vi "smu-dmm-test.vi"() -> ()   [LabVIEW 2020]
uses:
  Realization/NI DMM/NI DMM.lvclass
  Realization/NI DMM/TypeDefs/DMM waveform settings.ctl
  <instrlib>/niDMM/nidmm.llb/niDMM Waveform Function.ctl
  Realization/NI DMM/TypeDefs/Trigger settings.ctl
  <instrlib>/niDMM/nidmm.llb/niDMM Trigger.ctl
  <instrlib>/niDMM/nidmm.llb/niDMM Slope.ctl
  Realization/PIPX40 Relay/PIPX40 Relay.lvclass
  Realization/PIPX40 Matrix/PIPX40 Matrix.lvclass
  <instrlib>/niDCPower/nidcpower.llb/niDCPower Source Mode.ctl
  <instrlib>/niDCPower/nidcpower.llb/niDCPower Wait For Event - Event.ctl
  <instrlib>/niDCPower/nidcpower.llb/niDCPower Output Function.ctl
panel:
  in  "current limit range":dbl=0.01 format="%.6p"
  in  "voltage level range":dbl=6.0 format="%.6p"
  in  "current limit":dbl=0.01 format="%.6p"
  in  "voltage level":dbl=2.0 format="%.6p"
  in  "Source:Advanced:Source Delay":dbl=0.1
  out "Voltage Measurement":dbl
  out "Current Measurement":dbl
  out "Compliance/Limit Reached":bool
  in  "Channel Name":string="0"
  in  "Resource Name":refnum<k15>="NI_SMU1"
  out "relay info":variant
  out "Waveform Graph":dynamicdata(graph)
  out "error out":errorcluster
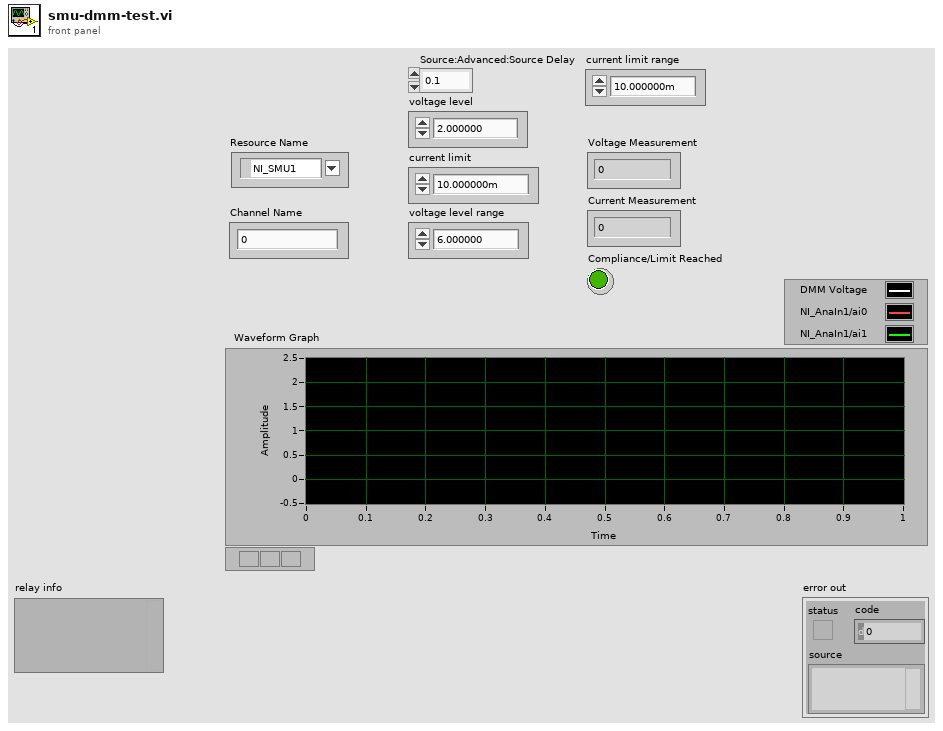
[diagram p1: front panel]
types:
  T1 = typedef "niDCPower Output Function.ctl" = i32
  T2 = typedef "niDCPower Wait For Event - Event.ctl" = i32
  T3 = typedef "niDCPower Source Mode.ctl" = i32
  T4 = typedef "NI DMM.lvlib/NI DMM.lvclass/Trigger settings.ctl" = cluster{"Trigger Source":T5, "Trigger Delay (sec)":dbl, "Slope":T6}
  T5 = typedef "niDMM Trigger.ctl" = enum16{"Immediate", "External", "TTL 0", "TTL 1", "TTL 2", "TTL 3", "TTL 4", "TTL 5", "TTL 6", "Software", "TTL 7", "PXI Star", "LBR Trig 1", "Aux Trig 1"}
  T6 = typedef "niDMM Slope.ctl" = enum16{"Rising Edge", "Falling Edge"}
  T7 = typedef "NI DMM.lvlib/NI DMM.lvclass/DMM waveform settings.ctl" = cluster{"Waveform Points":i32, "Function":T8, "Rate":dbl, "Range":dbl, "Settle Time":dbl}
  T8 = typedef "niDMM Waveform Function.ctl" = i32
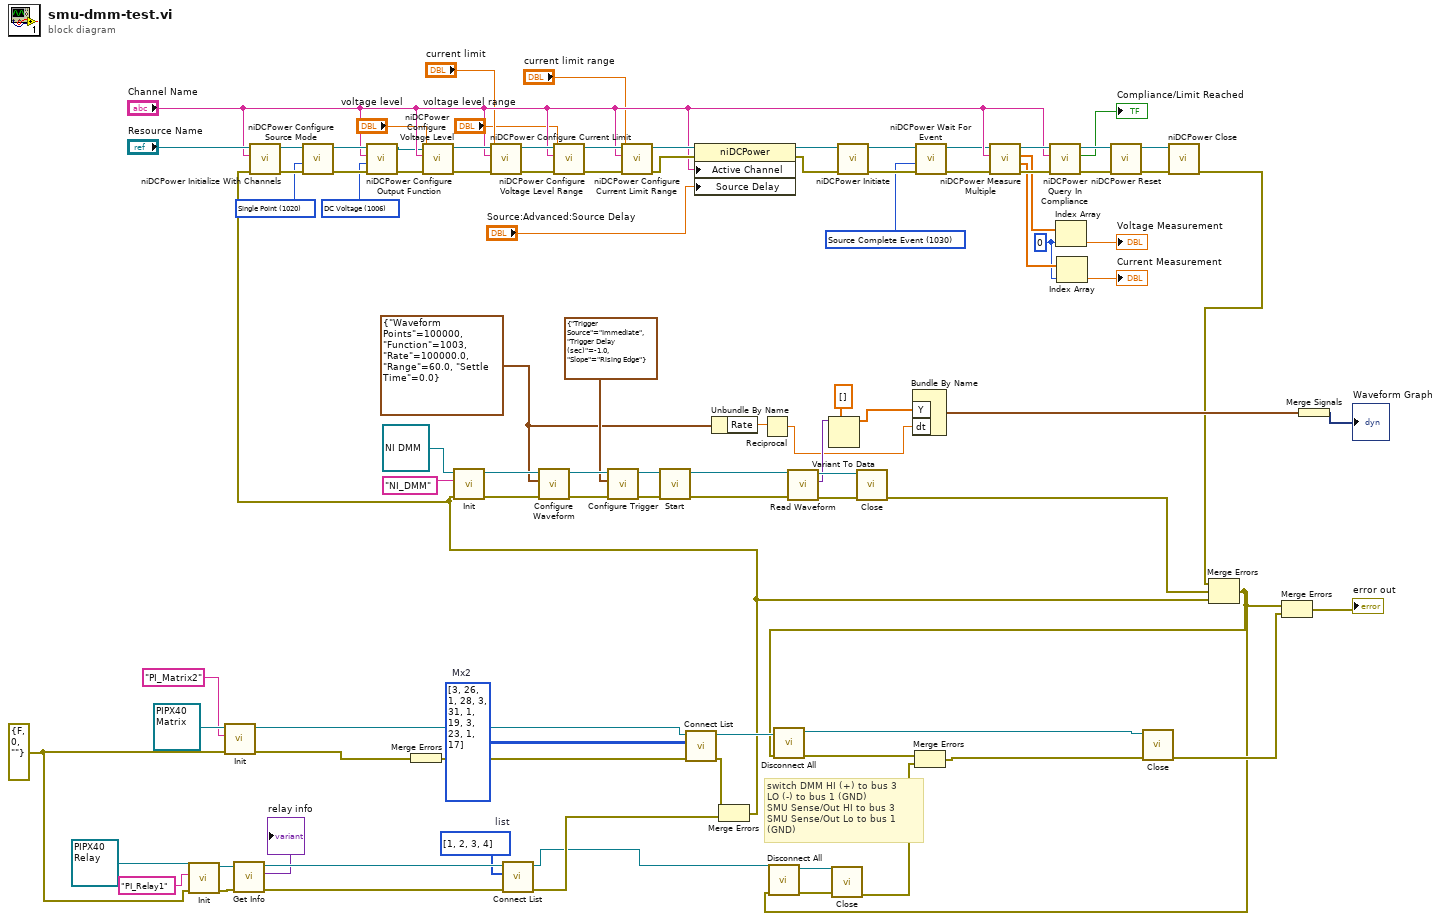
[diagram p0: block diagram]
diagram:
  w12 = T1 1006 items=["DC Voltage"=1006, "DC Current"=1007, "Pulse Voltage"=1049, "Pulse Current"=1050] ("output function")
  w16 = T2 1030 items=["Source Complete Event"=1030, "Measure Complete Event"=1031, "Sequence Iteration Complete Event"=1032, "Sequence Engine Done Event"=1033] ("event")
  w28 = 0 ("index")
  w37 = T3 1020 items=["Single Point"=1020, "Sequence"=1021] ("source mode")
  w59 = i32[] [1, 2, 3, 4]  # list
  w73 = T7 {"Waveform Points"=100000, "Function"=1003, "Rate"=100000.0, "Range"=60.0, "Settle Time"=0.0}
  w58 = errorcluster {"status"=FALSE, "code"=0, "source"=""} ("error in (no error)")
  w93 = i32[][] [[3, 26], [1, 28], [3, 31], [1, 19], [3, 23], [1, 17]]  # Mx2
  # "switch DMM HI (+) to bus 3 \nLO (-) to bus 1 (GND)\nSMU Sense/Out HI to bus 3\nSMU Sense/Out Lo to bus 1 (GND)"
  n1 = call-dynamic "Init.vi"("error in (no error)"=w58, "Params"="PI_Relay1" ("String"), "PIPXI40 Base in"=refnum<class "PIPX40 Relay.lvclass"> refnum ("Pickering.lvlib:PIPX40 Relay.lvclass")) -> ("error out"=w68:errorcluster, "PIPXI40 Base out"=w65:refnum<class "PIPX40 Relay.lvclass">)  [unwired: 7 in]
  n2 = call-dynamic "Init.vi"("error in (no error)"=w58, "Params"="PI_Matrix2" ("String"), "PIPXI40 Base in"=refnum<class "PIPX40 Matrix.lvclass"> refnum ("PIPXI40 Matrix in")) -> ("error out"=w53:errorcluster, "PIPXI40 Base out"=w51:refnum<class "PIPX40 Matrix.lvclass">)  [unwired: 7 in]
  n3 = call-dynamic "Get Info.vi"("error in (no error)"=w68, "PIPXI40 Base in"=w65) -> ("error out"=w62:errorcluster, "Info"=→"relay info":variant, "PIPXI40 Base out"=w64:refnum<class "PIPX40 Relay.lvclass">)  [unwired: 7 in]
  n4 = Merge Errors(w53) -> (w86:errorcluster)
  n5 = call-dynamic "Connect List.vi"("error in (no error)"=w62, "Params"=w59, "PIPXI40 Switching in"=w64) -> ("error out"=w55:errorcluster, "PIPXI40 Switching out"=w54:refnum<class "PIPX40 Relay.lvclass">)  [unwired: 7 in]
  n6 = call-dynamic "Connect List.vi"("error in (no error)"=w86, "Params"=w93, "PIPXI40 Matrix in"=w51) -> ("error out"=w89:errorcluster, "PIPXI40 Matrix out"=w92:refnum<class "PIPX40 Matrix.lvclass">)  [unwired: 7 in]
  n7 = Unbundle By Name(w73) -> ("Rate"=w72:dbl)
  n8 = Merge Errors(w89, w55) -> (w1:errorcluster)
  n9 = call <instrlib>:"niDCPower Initialize With Channels.vi"("error in (no error)"=w1, "channels"="Channel Name", "resource name"="Resource Name") -> ("error out"=w41:errorcluster, "instrument handle out"=w40:refnum<k15>)  [unwired: 2 in, 5 out]
  n10 = call <instrlib>:"niDCPower Configure Source Mode.vi"("error in (no error)"=w41, "source mode"=w37, "instrument handle"=w40) -> ("error out"=w39:errorcluster, "instrument handle out"=w38:refnum<k15>)  [unwired: 7 out]
  n11 = call <instrlib>:"niDCPower Configure Output Function.vi"("error in (no error)"=w39, "output function"=w12, "channel name"="Channel Name", "instrument handle"=w38) -> ("error out"=w14:errorcluster, "instrument handle out"=w15:refnum<k15>)  [unwired: 6 out]
  n12 = call <instrlib>:"niDCPower Configure Voltage Level.vi"("error in (no error)"=w14, "voltage level"="voltage level", "channel name"="Channel Name", "instrument handle"=w15) -> ("error out"=w46:errorcluster, "instrument handle out"=w47:refnum<k15>)  [unwired: 6 out]
  n13 = call-dynamic "Init.vi"("error in (no error)"=w1, "Params"="NI_DMM", "NI DMM in"=refnum<class "NI DMM.lvclass"> refnum) -> ("error out"=w84:errorcluster, "NI DMM out"=w85:refnum<class "NI DMM.lvclass">)  [unwired: 7 in]
  n14 = call <instrlib>:"niDCPower Configure Current Limit.vi"("error in (no error)"=w46, "current limit"="current limit", "channel name"="Channel Name", "instrument handle"=w47) -> ("error out"=w36:errorcluster, "instrument handle out"=w35:refnum<k15>)  [unwired: 1 in, 5 out]
  n15 = call-dynamic "Configure Waveform.vi"("error in (no error)"=w84, "Params"=w73, "NI DMM in"=w85) -> ("error out"=w80:errorcluster, "NI DMM out"=w81:refnum<class "NI DMM.lvclass">)  [unwired: 7 in]
  n16 = call <instrlib>:"niDCPower Configure Voltage Level Range.vi"("error in (no error)"=w36, "voltage level range"="voltage level range", "channel name"="Channel Name", "instrument handle"=w35) -> ("error out"=w34:errorcluster, "instrument handle out"=w33:refnum<k15>)  [unwired: 6 out]
  n17 = call-dynamic "Configure Trigger.vi"("error in (no error)"=w80, "Params"=T4 {"Trigger Source"=enum."Immediate", "Trigger Delay (sec)"=-1.0, "Slope"=enum."Rising Edge"}, "NI DMM in"=w81) -> ("error out"=w5:errorcluster, "NI DMM out"=w4:refnum<class "NI DMM.lvclass">)  [unwired: 7 in]
  n18 = call <instrlib>:"niDCPower Configure Current Limit Range.vi"("error in (no error)"=w34, "current limit range"="current limit range", "channel name"="Channel Name", "instrument handle"=w33) -> ("error out"=w22:errorcluster, "instrument handle out"=w25:refnum<k15>)  [unwired: 6 out]
  n19 = call-dynamic "Start.vi"("error in (no error)"=w5, "DMM in"=w4) -> ("error out"=w2:errorcluster, "DMM out"=w3:refnum<class "NI DMM.lvclass">)  [unwired: 8 in]
  n20 = property class="niDCPower"(reference=w25, error in=w22, "Active Channel"="Channel Name", "Source Delay"="Source:Advanced:Source Delay") -> (reference out=w24:refnum<k15>, error out=w23:errorcluster)
  n21 = Reciprocal(x=w72) -> (1/x=w71:dbl)
  n22 = call-dynamic "Read Waveform.vi"("error in (no error)"=w2, "NI DMM in"=w3) -> ("error out"=w78:errorcluster, "Data"=w76:variant, "NI DMM out"=w77:refnum<class "NI DMM.lvclass">)  [unwired: 7 in]
  n23 = Variant To Data(type=dbl[] [], Variant=w76) -> (data=w74:dbl[])  [unwired: 1 in, 1 out]
  n24 = call <instrlib>:"niDCPower Initiate.vi"("error in (no error)"=w23, "instrument handle"=w24) -> ("error out"=w18:errorcluster, "instrument handle out"=w20:refnum<k15>)  [unwired: 2 in, 6 out]
  n25 = call-dynamic "Close.vi"("error in (no error)"=w78, "NI DMM in"=w77) -> ("error out"=w69:errorcluster)  [unwired: 8 in, 1 out]
  n26 = Bundle By Name("Y"=w74, "dt"=w71) -> (w70:waveform(dbl))  [unwired: 1 in]
  n27 = call <instrlib>:"niDCPower Wait For Event.vi"("error in (no error)"=w18, "event"=w16, "instrument handle"=w20) -> ("error out"=w17:errorcluster, "instrument handle out"=w19:refnum<k15>)  [unwired: 1 in, 6 out]
  n28 = call <instrlib>:"niDCPower Measure Multiple.vi"("error in (no error)"=w17, "channel name"="Channel Name", "instrument handle"=w19) -> ("error out"=w31:errorcluster, "current measurements"=w29:dbl[], "voltage measurements"=w30:dbl[], "instrument handle out"=w32:refnum<k15>)  [unwired: 5 out]
  n29 = call <instrlib>:"niDCPower Query In Compliance.vi"("error in (no error)"=w31, "channel name"="Channel Name", "instrument handle"=w32) -> ("error out"=w42:errorcluster, "in compliance?"=→"Compliance/Limit Reached":bool, "instrument handle out"=w45:refnum<k15>)  [unwired: 6 out]
  n30 = Index Array(array=w30, index=w28) -> (element=→"Voltage Measurement":dbl)
  n31 = Index Array(array=w29, index=w28) -> (element=→"Current Measurement":dbl)
  n32 = call <instrlib>:"niDCPower Reset.vi"("error in (no error)"=w42, "instrument handle"=w45) -> ("error out"=w43:errorcluster, "instrument handle out"=w44:refnum<k15>)  [unwired: 2 in, 6 out]
  n33 = call <instrlib>:"niDCPower Close.vi"("error in (no error)"=w43, "instrument handle"=w44) -> ("error out"=w11:errorcluster)  [unwired: 9 out]
  n34 = Merge Errors(w11, w69, w1) -> (w57:errorcluster)
  n35 = call-dynamic "Disconnect All.vi"("error in (no error)"=w57, "PIPXI40 Switching in"=w54) -> ("error out"=w60:errorcluster, "PIPXI40 Switching out"=w61:refnum<class "PIPX40 Relay.lvclass">)  [unwired: 8 in]
  n36 = call-dynamic "Disconnect All.vi"("error in (no error)"=w57, "PIPXI40 Matrix in"=w92) -> ("error out"=w91:errorcluster, "PIPXI40 Matrix out"=w49:refnum<class "PIPX40 Matrix.lvclass">)  [unwired: 8 in]
  n37 = call-dynamic "Close.vi"("error in (no error)"=w60, "PIPXI40 Base in"=w61) -> ("error out"=w56:errorcluster)  [unwired: 8 in, 1 out]
  n38 = Merge Errors(w91, w56) -> (w90:errorcluster)
  n39 = call-dynamic "Close.vi"("error in (no error)"=w90, "PIPXI40 Base in"=w49) -> ("error out"=w88:errorcluster)  [unwired: 8 in, 1 out]
  n40 = Merge Errors(w57, w88) -> (→"error out":errorcluster)
  n41 = Merge Signals(w70) -> (→"Waveform Graph":dynamicdata)
